vi "PicoScope5000aExampleRapidBlock.vi"() -> ()   [LabVIEW 2016]
panel:
  in  "Serial Number":string
  in  "Open using Serial Number":bool
  in  "Resolution":i32(ring)=4 items=["8-bit", "12-bit", "14-bit", "15-bit (max. 2 ch.)", "16-bit (max. 1 ch.)"]
  in  "PS5X4XA/B\nUSB Powered":bool=TRUE
  in  "Trigger Settings":T1={"Trigger Enabled"=TRUE, "Trigger Source"=enum."Channel A", "Trigger Threshold (16-bit counts)"=16384, "Trigger Direction"=2, "Trigger Delay (samples)"=0, "Auto Trigger Time (ms)"=0} {"Trigger Direction" items=["Rising"=2, "Falling"=3]}
  in  "Channel A Settings":T2={"Enabled"=TRUE, "Coupling"=1, "Range"=6, "Analogue Offset"=0.0} {"Range" items=["10 mV", "20 mV", "50 mV", "100 mV", "200 mV", "500 mV", "1 V", "2 V", "5 V", "10 V", "20 V", "50 V ", "100 V"]; "Coupling" items=["AC", "DC"]}
  in  "Rapid Block Acquisition Settings":T3={"preTriggerSamples"=0, "postTriggerSamples"=1024, "timebase"=10, "Four Channel Device"=FALSE, "Number of Captures"=100}
  out "Capture Complete":bool
  in  "Run":bool
  out "Channel A":i16[][](graph)
  in  "Capture Index":i16 min=0
  in  "stop":bool
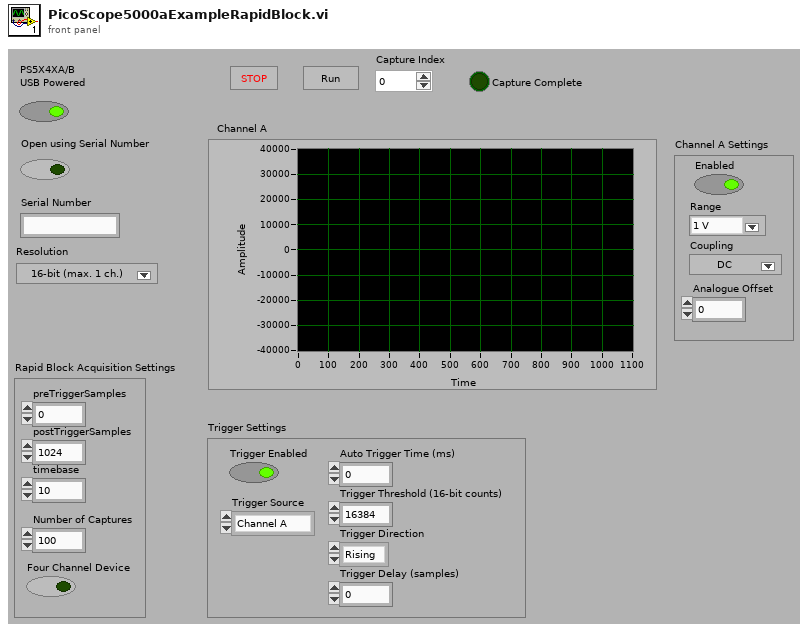
[diagram p1: front panel]
types:
  T1 = cluster{"Trigger Enabled":bool, "Trigger Source":enum16{"Channel A", "Channel B", "Channel C", "Channel D", "Ext."}, "Trigger Threshold (16-bit counts)":i16, "Trigger Direction":u16, "Trigger Delay (samples)":u32, "Auto Trigger Time (ms)":i16}
  T2 = cluster{"Enabled":bool, "Coupling":i16, "Range":u16, "Analogue Offset":sgl}
  T3 = cluster{"preTriggerSamples":u32, "postTriggerSamples":u32, "timebase":u32, "Four Channel Device":bool, "Number of Captures":u32}
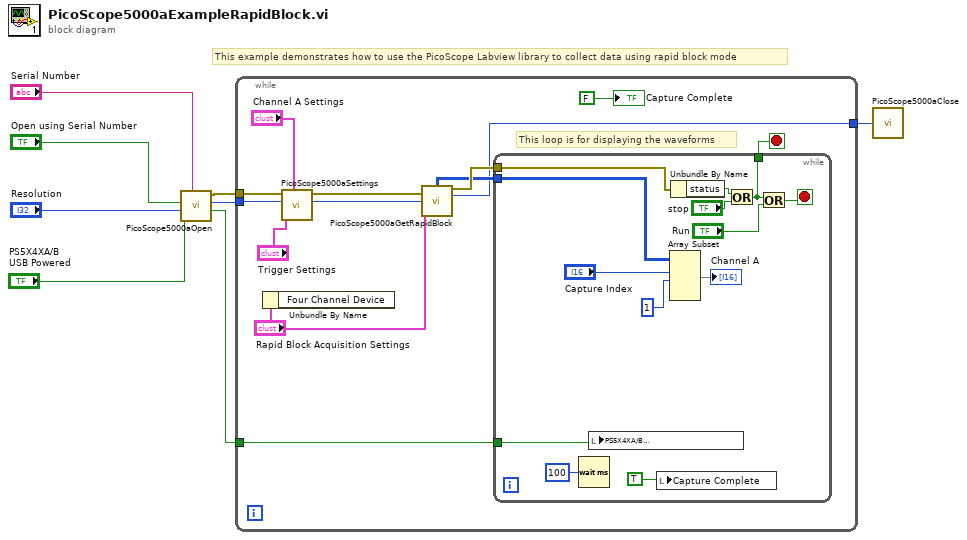
[diagram p0: block diagram]
diagram:
  # "This example demonstrates how to use the PicoScope Labview library to collect data using rapid block mode"
  n1 = call "PicoScope5000aOpen.vi"("Serial Number"="Serial Number", "USB Powered Selection"="PS5X4XA/B\nUSB Powered", "Resolution"="Resolution", "Use Serial Number"="Open using Serial Number") -> ("USB Powered Indication"=w4:bool, "handle"=w6:i16, "error out"=w7:errorcluster)  [unwired: 3 in, 2 out]
  n2 = while {
    tunnel: [w17] -> w8
    tunnel: w7 -> [w12]
    tunnel: w6 -> [w11]
    tunnel: w4 -> [w10]
    stop <- w21 stop-if-true
    # "This loop is for displaying the waveforms"
    n3 = Unbundle By Name("Rapid Block Acquisition Settings") -> ()  [unwired: 1 out]
    n4 = call "PicoScope5000aSettings.vi"("Channel A Settings"="Channel A Settings", "Trigger Settings"="Trigger Settings", "handle in"=w11, "error in"=w12) -> ("handle out"=w16:i16, "error out"=w15:errorcluster)  [unwired: 6 in]
    n5 = call "PicoScope5000aGetRapidBlock.vi"("error in"=w15, "handle in"=w16, "Rapid Block Acquisition Settings"="Rapid Block Acquisition Settings") -> ("Channel A Buffer"=w18:i16[][], "error out"=w19:errorcluster, "handle out"=w17:i16)  [unwired: 7 in, 3 out]
    n6 = while {
      tunnel: [w31] -> w21
      tunnel: w18 -> [w26]
      tunnel: w19 -> [w25]
      tunnel: w10 -> [w22]
      stop <- w30 stop-if-true
      n7 = Wait (ms)(milliseconds to wait=u32 100) -> ()  [unwired: 1 out]
      n8 = local write "PS5X4XA/B\nUSB Powered"(w22) -> ()
      n9 = local write "Capture Complete"(TRUE ("Capture Complete")) -> ()
      n10 = Array Subset(array=w26, index (row)="Capture Index", length (row)=1 ("length")) -> (→"Channel A":i16[][])  [unwired: 2 in]
      n11 = Unbundle By Name(w25) -> ("status"=w24:bool)
      n12 = Or(x=w24, y="stop") -> (x .or. y?=w31:bool)
      n13 = Or(x=w31, y="Run") -> (x .or. y?=w30:bool)
    }
    "Capture Complete" <- FALSE ("Capture Complete")
  }
  n14 = call "PicoScope5000aClose.vi"("handle"=w8) -> ()
